vi "SweepTemperatureStateMachine.vi"(0 "SweepTempState":T2(ring), 5 "SweepT":T1={"Temp Start"=0.0, "Temp Stop"=0.0, "Delta T"=0.5, "Dwell Time"=0.0, "Temp Tol"=0.5} {"Temp Tol" min=0.01 step=0.5 format="%.3f"; "Dwell Time" min=0.0 step=0.1 format="%.1f"; "Delta T" min=0.5 step=0.5 format="%.1f"; "Temp Stop" step=0.5 format="%.1f"; "Temp Start" step=0.5 format="%.1f"}, 7 "Filter Temp":dbl step=0.5 format="%.1f", 9 "Start New Sweep Ref":refnum<vi>, 11 "error in (no error)":errorcluster, 12 "start new profille":bool) -> (4 "SweepTempState out":T2(ring), 6 "Current Req Temp":dbl, 15 "error out":errorcluster)   [LabVIEW 2013]
doc: "Temperature sweep is implemented with a state machine pattern."
panel:
  out "Timer":dbl
  # "Input"
  # "output"
  # "°C"
  # "°C"
  # "°C"
  # "min"
  # "°C"
  # "°C"
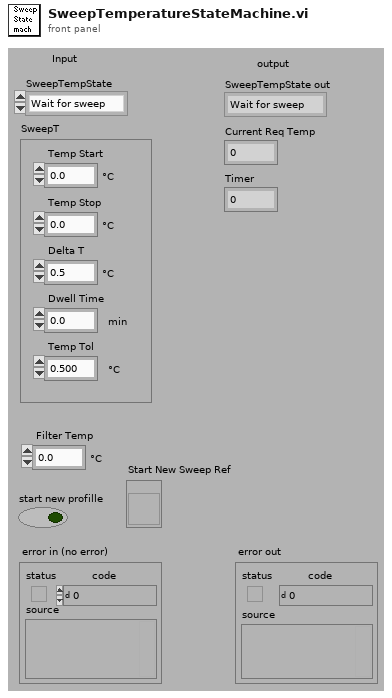
[diagram p1: front panel]
types:
  T1 = cluster{"Temp Start":dbl, "Temp Stop":dbl, "Delta T":dbl, "Dwell Time":dbl, "Temp Tol":dbl}
  T2 = enum16{"Wait for sweep", "Reaching Set Temp", "Wait at Temp"}
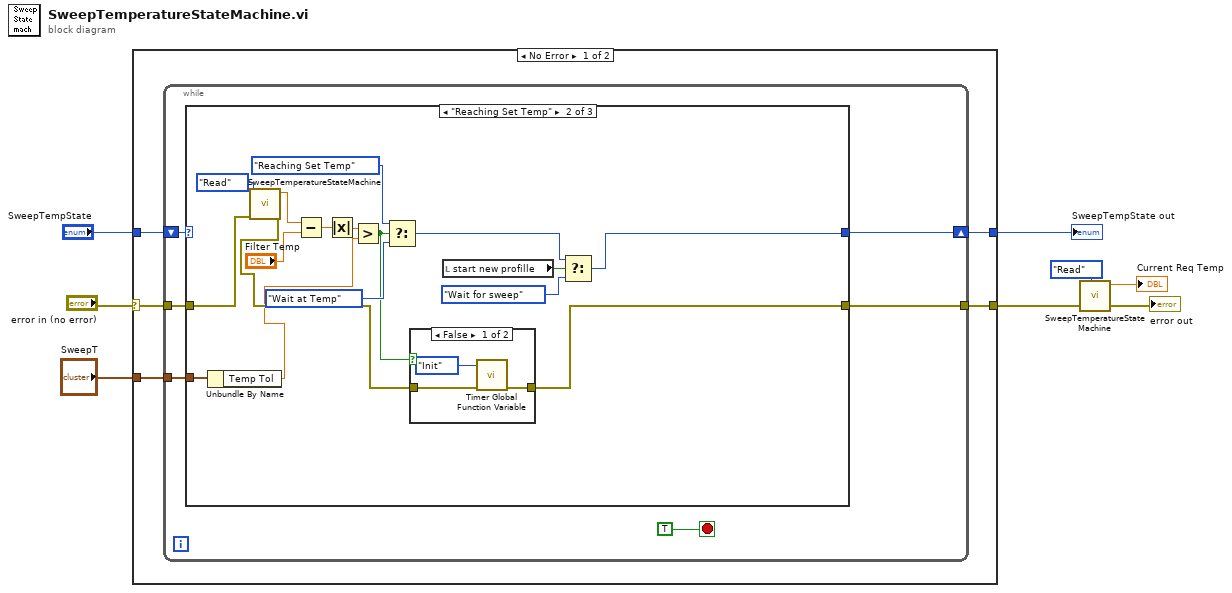
[diagram p0: block diagram]
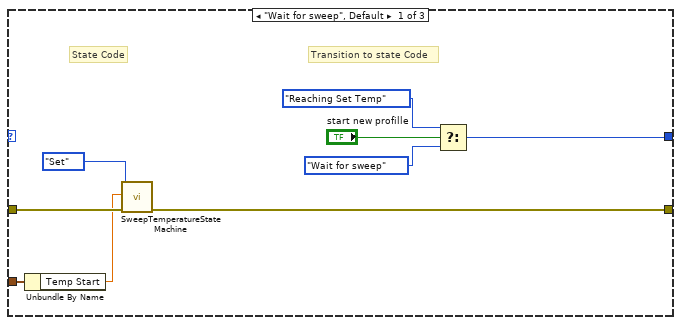
[diagram p2: hidden frame]
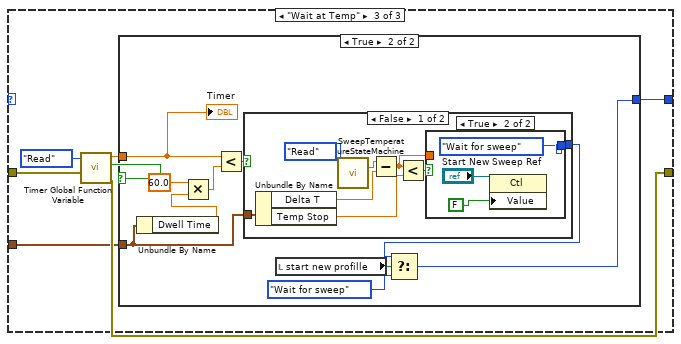
[diagram p4: hidden frame]
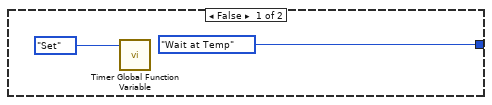
[diagram p5: hidden frame]
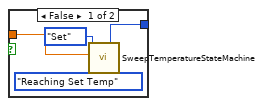
[diagram p6: hidden frame]
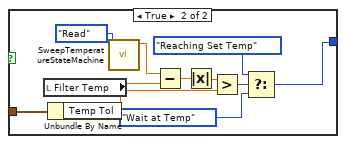
[diagram p7: hidden frame]
diagram:
  n1 = case shown="No Error" "error in (no error)" {
    selector: "error in (no error)" -> [w10 w94]
    tunnel: [w9 w94] -> w4
    tunnel: "SweepTempState" -> [w12 w93]
    tunnel: [w11 w93] -> w5
    tunnel: "SweepT" -> [w8 _]
    frame No Error {
      n2 = while {
        shift-right: [w17] -> w11
        shift-left: w12 -> [w15]
        tunnel: w10 -> [w16]
        tunnel: [w14] -> w9
        tunnel: w8 -> [w13]
        stop <- TRUE stop-if-true
        n3 = case shown="\"Reaching Set Temp\"" w15 {
          tunnel: [w25 w33 w52] -> w17
          tunnel: w16 -> [w22 w43 w51]
          tunnel: [w21 w30 w50] -> w14
          tunnel: w13 -> [w20 w29 w49]
          frame "Wait for sweep", Default {
            # "State Code"
            # "Transition to state Code"
            n4 = Unbundle By Name(w20) -> ("Temp Start"=w19:dbl)
            n5 = call "SweepTemperatureStateMachine.vi"("error in (no error)"=w22, "Request Temperature"=w19, "Enum"=enum16{"Init", "Read", "Set"}."Set") -> ("error out"=w21:errorcluster)  [unwired: 6 in, 2 out]
            n6 = Select(t=T2."Reaching Set Temp" ("SweepTempState"), s="start new profille", f=T2."Wait for sweep" ("SweepTempState")) -> (s? t:f=w25:T2)
          }
          frame "Reaching Set Temp" {
            n7 = Unbundle By Name(w29) -> ("Temp Tol"=w28:dbl)
            n8 = call "SweepTemperatureStateMachine.vi"("error in (no error)"=w43, "Enum"=enum16{"Init", "Read", "Set"}."Read") -> ("error out"=w31:errorcluster, "Current Req Temp"=w42:dbl)  [unwired: 7 in, 1 out]
            n9 = Subtract(x=w42, y="Filter Temp") -> (x-y=w40:dbl)
            n10 = Absolute Value(x=w40) -> (abs(x)=w39:dbl)
            n11 = Greater?(x=w39, y=w28) -> (0:w32:bool)
            n12 = Select(t=T2."Reaching Set Temp" ("SweepTempState"), s=w32, f=T2."Wait at Temp" ("SweepTempState")) -> (s? t:f=w34:T2)
            n13 = case shown="False" w32 {
              tunnel: w31 -> [w46 w48]
              tunnel: [w45 w48] -> w30
              frame False {
                n14 = call "Timer Global Function Variable.vi"("error in (no error)"=w46, "Enum"=enum16{"Init", "Read", "Set"}."Init") -> ("error out"=w45:errorcluster)  [unwired: 7 in, 2 out]
              }
              frame True {
              }
            }
            n15 = local read "start new profille"() -> (w36:bool)
            n16 = Select(t=w34, s=w36, f=T2."Wait for sweep" ("SweepTempState")) -> (s? t:f=w33:T2)
          }
          frame "Wait at Temp" {
            n17 = call "Timer Global Function Variable.vi"("error in (no error)"=w51, "Enum"=enum16{"Init", "Read", "Set"}."Read") -> ("error out"=w50:errorcluster, "Timer Counting"=w54:bool, "Time Elapsed"=w53:dbl)  [unwired: 7 in]
            n18 = case shown="True" w54 {
              tunnel: w53 -> [_ w61]
              tunnel: [T2."Wait at Temp" ("SweepTempState") w64] -> w52
              tunnel: w49 -> [_ w60]
              frame False {
                n19 = call "Timer Global Function Variable.vi"("Enum"=enum16{"Init", "Read", "Set"}."Set") -> ()  [unwired: 8 in, 3 out]
              }
              frame True {
                n20 = Unbundle By Name(w60) -> ("Dwell Time"=w59:dbl)
                n21 = Multiply(x=60.0 ("y"), y=w59) -> (x*y=w67:dbl)
                n22 = Less?(x=w61, y=w67) -> (x < y?=w63:bool)
                n23 = case shown="False" w63 {
                  tunnel: [w71 w84] -> w62
                  tunnel: w60 -> [w70 w82]
                  frame False {
                    n24 = Unbundle By Name(w70) -> ("Delta T"=w69:dbl, "Temp Stop"=w68:dbl)
                    n25 = call "SweepTemperatureStateMachine.vi"("SweepTempState"=enum16{"Init", "Read", "Set"}."Read" ("Enum")) -> ("Current Req Temp"=w74:dbl)  [unwired: 12 in, 2 out]
                    n26 = Subtract(x=w74, y=w69) -> (x-y=w72:dbl)
                    n27 = Less?(x=w72, y=w68) -> (x < y?=w73:bool)
                    n28 = case shown="True" w73 {
                      tunnel: w72 -> [w77 _]
                      tunnel: [T2."Reaching Set Temp" ("SweepTempState") T2."Wait for sweep" ("SweepTempState")] -> w71
                      frame False {
                        n29 = call "SweepTemperatureStateMachine.vi"("Request Temperature"=w77, "Enum"=enum16{"Init", "Read", "Set"}."Set") -> ()  [unwired: 7 in, 3 out]
                      }
                      frame True {
                        n30 = property class="Ctl"(reference="Start New Sweep Ref", "Value"=FALSE) -> ()  [unwired: 1 in, 2 out]
                      }
                    }
                  }
                  frame True {
                    n31 = local read "Filter Temp"() -> (w86:dbl)
                    n32 = Unbundle By Name(w82) -> ("Temp Tol"=w83:dbl)
                    n33 = call "SweepTemperatureStateMachine.vi"("Enum"=enum16{"Init", "Read", "Set"}."Read") -> ("Current Req Temp"=w91:dbl)  [unwired: 8 in, 2 out]
                    n34 = Subtract(x=w91, y=w86) -> (x-y=w90:dbl)
                    n35 = Absolute Value(x=w90) -> (abs(x)=w89:dbl)
                    n36 = Greater?(x=w89, y=w83) -> (0:w87:bool)
                    n37 = Select(t=T2."Reaching Set Temp" ("SweepTempState"), s=w87, f=T2."Wait at Temp" ("SweepTempState")) -> (s? t:f=w84:T2)
                  }
                }
                n38 = local read "start new profille"() -> (w66:bool)
                n39 = Select(t=w62, s=w66, f=T2."Wait for sweep" ("SweepTempState")) -> (s? t:f=w64:T2)
                "Timer" <- w61
              }
            }
          }
        }
      }
    }
    frame Error {
    }
  }
  "error out" <- w4
  "SweepTempState out" <- w5
  n40 = call "SweepTemperatureStateMachine.vi"("Enum"=enum16{"Init", "Read", "Set"}."Read") -> ("Current Req Temp"=→"Current Req Temp":dbl)  [unwired: 8 in, 2 out]
